vi "Add Modules.vi"(8 "error in (no error)":errorcluster, 10 "Modules":T1[](array[typedef]), 11 "Block Diagram in":refnum<class "VI.lvclass">) -> (0 "error out":errorcluster, 3 "Block Diagram out":refnum<class "VI.lvclass">)   [LabVIEW 2025, in "VI.lvclass"]
doc: "Script all the required code for the signal IP."
uses:
  VI.lvclass
  Module/Module/Module Settings.ctl
  Signal/Signal/Signal Settings.ctl
  VI.lvclass/VI.ctl
  BlockDiagram.Refs.ctl
  Module.Refs.ctl
  <vilib>/Utility/miscctls.llb/LVPointTypeDef.ctl
  Module Loop/Module Loop.lvclass
  Structures/Read Diagram.vi
  Structures/Read Location.vi
  Module Loop/Read EST Tunnel.vi
  Module/Module/Module.lvclass
  DMA Loop/DMA Loop.lvclass
  Signal/Signal/Signal.lvclass
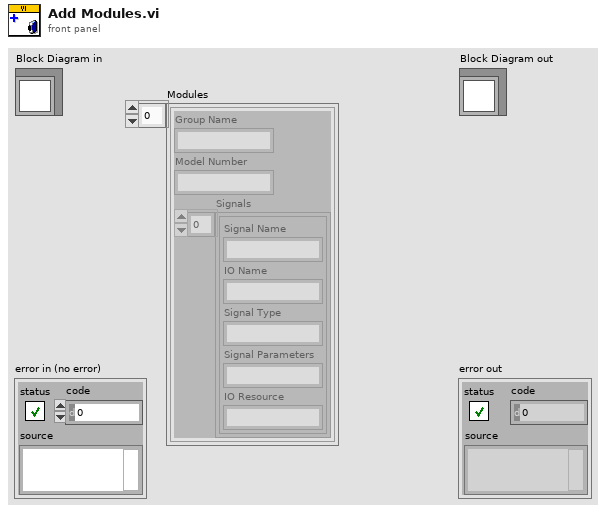
[diagram p1: front panel]
types:
  T1 = typedef "Module.lvclass/Module Settings.ctl" = cluster{"Group Name":string, "Model Number":string, "Signals":T2[]}
  T2 = typedef "Signal.lvclass/Signal Settings.ctl" = cluster{"Signal Name":string, "IO Name":string, "Signal Type":string, "Signal Parameters":string, "IO Resource":string}
  T3 = typedef "VI.lvclass/BlockDiagram.Refs.ctl" = cluster{"Top.Diagram":refnum<vi>, "ModuleLoop":T4}
  T4 = typedef "VI.lvclass/Module.Refs.ctl" = cluster{"Diagram":refnum<vi>, "Location":refnum<data-value>, "ESTTunnel":refnum<vi>}
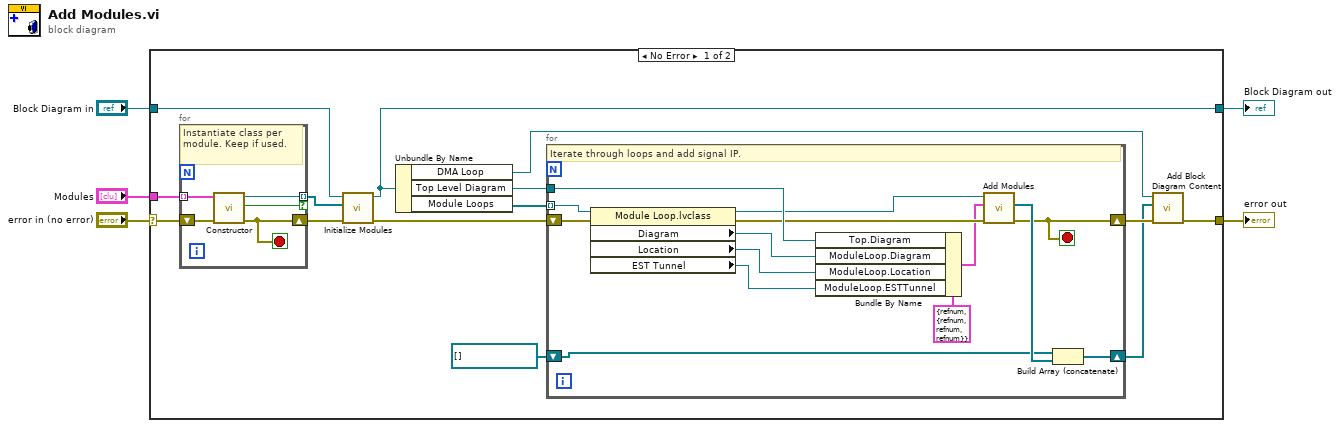
[diagram p0: block diagram]
diagram:
  n1 = case shown="No Error" "error in (no error)" {
    selector: "error in (no error)" -> [w8 w40]
    tunnel: [w12 w40] -> w4
    tunnel: [w14 w39] -> w2
    tunnel: "Block Diagram in" -> [w15 w39]
    tunnel: "Modules" -> [w9 _]
    frame No Error {
      n2 = for {
        tunnel: w9 -> [w24] mode=indexing
        shift-right: [w20] -> w6
        shift-left: w8 -> [w23]
        tunnel: [w22] -> w7 mode=indexing if=w21
        stop <- w20 stop-if-true
        # "Instantiate class per module. Keep if used."
        n3 = call "Constructor.vi"("error in (no error)"=w23, "Module Settings"=w24) -> ("error out"=w20:errorcluster, "Use?"=w21:bool, "Module.lvclass"=w22:refnum<class "Module.lvclass">)  [unwired: 7 in]
      }
      n4 = call "Initialize Modules.vi"("error in (no error)"=w6, "Modules"=w7, "Block Diagram in"=w15) -> ("error out"=w16:errorcluster, "Block Diagram out"=w14:refnum<class "VI.lvclass">)  [unwired: 7 in]
      n5 = Unbundle By Name(w14) -> ("DMA Loop"=w11:refnum<class "DMA Loop.lvclass">, "Top Level Diagram"=w18:refnum<vi>, "Module Loops"=w19:refnum<class "Module Loop.lvclass">[])
      n6 = for {
        shift-right: [w25] -> w13
        shift-left: w16 -> [w38]
        tunnel: w19 -> [w37] mode=indexing
        tunnel: w18 -> [w36]
        shift-right: [w27] -> w10
        shift-left: refnum<vi>[] [] -> [w26]
        stop <- w25 stop-if-true
        # "Iterate through loops and add signal IP."
        n7 = property class="Module Loop.lvclass"(reference=w37, error in=w38) -> (reference out=w31:refnum<class "Module Loop.lvclass">, error out=w30:errorcluster, "Diagram"=w35:refnum<vi>, "Location"=w34:refnum<data-value>, "EST Tunnel"=w33:refnum<vi>)
        n8 = Bundle By Name(cluster=T3 {"Top.Diagram"=refnum, "ModuleLoop"={"Diagram"=refnum, "Location"=refnum, "ESTTunnel"=refnum}}, "Top.Diagram"=w36, "ModuleLoop.Diagram"=w35, "ModuleLoop.Location"=w34, "ModuleLoop.ESTTunnel"=w33) -> (w29:T3)
        n9 = call-dynamic "Add Modules.vi"("error in (no error)"=w30, "Refs"=w29, "IO Loop in"=w31) -> ("error out"=w25:errorcluster, "Mod.Locals.Ref"=w28:refnum<vi>[])  [unwired: 6 in, 1 out]
        n10 = Build Array (concatenate)(w26, w28) -> (w27:refnum<vi>[])
      }
      n11 = call "Add Block Diagram Content.vi"("error in (no error)"=w13, "Mod.Locals.Ref"=w10, "DMA Loop in"=w11) -> ("error out"=w12:errorcluster)  [unwired: 7 in, 1 out]
    }
    frame Error {
    }
  }
  "error out" <- w4
  "Block Diagram out" <- w2
